vi "Q Vision_2017 Object Calcs.vi"(4 "Threshhold":i32=50, 6 "ColorMask Low/High":u8[][](array[numeric])=[[0, 100], [200, 255], [170, 230]], 7 "ColorSpace":T1, 8 "error in (no error)":errorcluster, 10 "Image in":T3) -> (0 "error out":errorcluster, 3 "Object Params out":T2 {"Deg_Up" format="%.2f"; "Deg_Rt" format="%.2f"; "Dist_ft" format="%.1f"})   [LabVIEW 2016]
uses:
  <vilib>/vision/Image Controls.llb/IMAQ Image.ctl
  Typedefs/typedef_cluster_Object Params.ctl
  Quick Vision/Typedefs/typedef_enum_ColorSpace.ctl
panel:
  out "B/W Image":i16[][](graph)
  out "Image Pixels (U32)":u32[][](array[numeric]) format="%08x"
  out "B/W Image_Object":i16[][](graph)
  # "R"
  # "G"
  # "B"
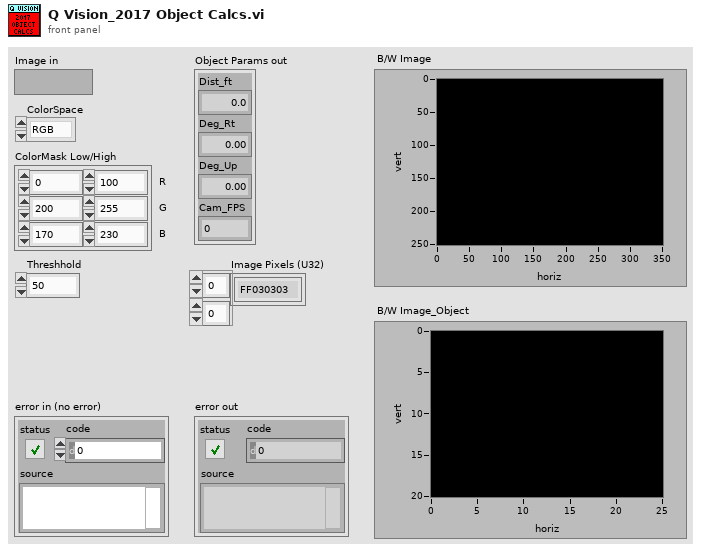
[diagram p1: front panel]
types:
  T1 = typedef "typedef_enum_ColorSpace.ctl" = enum16{"RGB", "HSL"}
  T2 = typedef "typedef_cluster_Object Params.ctl" = cluster{"Dist_ft":dbl, "Deg_Rt":dbl, "Deg_Up":dbl, "Cam_FPS":dbl}
  T3 = typedef "IMAQ Image.ctl" = refnum<image>
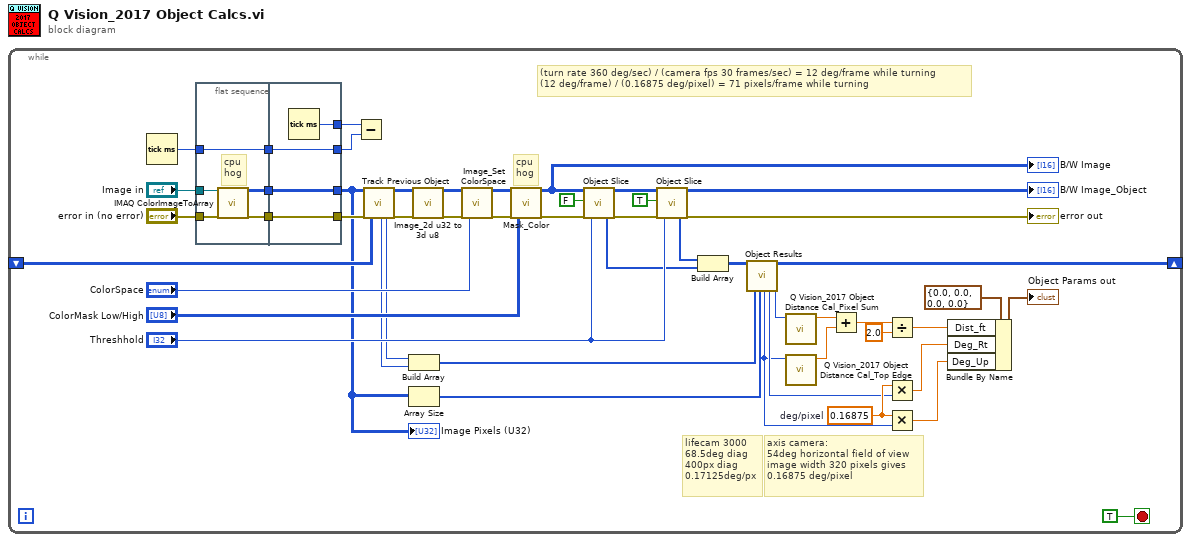
[diagram p0: block diagram]
diagram:
  n1 = while {
    shift-right: [w12] -> _
    shift-left: _ -> [w23]
    stop <- TRUE stop-if-true
    w31 = 0.16875  # deg/pixel
    # "lifecam 3000\n68.5deg diag\n400px diag\n0.17125deg/px"
    # "(turn rate 360 deg/sec) / (camera fps 30 frames/sec) = 12 deg/frame while turning\n(12 deg/frame) / (0.16875 deg/pixel) = 71 pixels/frame while turning"
    # "axis camera:\n54deg horizontal field of view\nimage width 320 pixels gives\n0.16875 deg/pixel"
    # "cpu\nhog"
    n2 = Tick Count (ms)() -> (millisecond timer value=w39:u32)
    n3 = flat-sequence {
      tunnel: [w55] -> w49
      tunnel: [w53] -> w48
      tunnel: [w54] -> w47
      tunnel: w39 -> [w53]
      tunnel: "Image in" -> [w52]
      tunnel: "error in (no error)" -> [w51]
      tunnel: [w57] -> w22
      tunnel: [w58] -> w33
      tunnel: [w59] -> w20
      tunnel: w49 -> [w59]
      tunnel: w48 -> [w58]
      tunnel: w47 -> [w57]
      tunnel: [w56] -> w34
      frame #0 {
        # "cpu\nhog"
        n4 = call "IMAQ ColorImageToArray"("Image"=w52, "error in (no error)"=w51) -> ("Image Pixels (U32)"=w55:u32[][], "error out"=w54:errorcluster)  [unwired: 2 in, 1 out]
      }
      frame #1 {
        n5 = Tick Count (ms)() -> (millisecond timer value=w56:u32)
      }
    }
    n6 = Subtract(x=w34, y=w33) -> ()  [unwired: 1 out]
    n7 = call "Track Previous Object.vi"("Image_2d_u32 in"=w20, "error in (no error)"=w22, "Prev. Object Start/Stop/Sum"=w23) -> ("Col Offset"=w17:i32, "Row Offset"=w18:i32, "Image_2d_u32 out"=w24:u32[][], "error out"=w21:errorcluster)  [unwired: 13 in]
    n8 = Build Array(w18, w17) -> (w8:i32[])
    n9 = Array Size(array=w20) -> (size(s)=w9:i32[])
    n10 = call "Image_2d u32 to 3d u8.vi"("Image_2d_u32"=w24, "error in (no error)"=w21) -> ("Image_3d_u8"=w45:u8[][][], "error out"=w43:errorcluster)  [unwired: 16 in]
    n11 = call "Image_Set ColorSpace.vi"("Image_3d"=w45, "error in (no error)"=w43, "ColorSpace"="ColorSpace") -> ("Image_3d_ColorSpace"=w44:u8[][][], "error out"=w46:errorcluster)  [unwired: 14 in, 1 out]
    n12 = call "Mask_Color.vi"("Image_3d"=w44, "error in (no error)"=w46, "ColorMask Low/High"="ColorMask Low/High") -> ("Image_2d"=w30:i16[][], "error out"=w42:errorcluster)  [unwired: 14 in, 1 out]
    "B/W Image" <- w30
    n13 = call "Object Slice.vi"("Image_2d"=w30, "Slice Rows(T)/Cols(F)"=FALSE, "error in (no error)"=w42, "Threshhold"="Threshhold") -> ("Object Start/Stop/Sum"=w15:i32[], "Image_2d_Slice"=w40:i16[][], "error out"=w27:errorcluster)  [unwired: 13 in]
    n14 = call "Object Slice.vi"("Image_2d"=w40, "Slice Rows(T)/Cols(F)"=TRUE, "error in (no error)"=w27, "Threshhold"="Threshhold") -> ("Object Start/Stop/Sum"=w16:i32[], "Image_2d_Slice"=→"B/W Image_Object":i16[][], "error out"=→"error out":errorcluster)  [unwired: 13 in]
    n15 = Build Array(w16, w15) -> (w13:i32[][])
    n16 = call "Object Results.vi"("Object Start/Stop/Sum in"=w13, "Offset rows,cols"=w8, "Image rows,cols"=w9) -> ("Pixels Up"=w5:i32, "Pixels Rt"=w10:i32, "Object Start/Stop/Sum out"=w12:i32[][], "Pixel Sum"=w11:i32)  [unwired: 13 in]
    n17 = call "Q Vision_2017 Object Distance Cal_Pixel Sum.vi"("Pixel Sum"=w11) -> ("Distance (ft)"=w6:dbl)  [unwired: 10 in]
    n18 = call "Q Vision_2017 Object Distance Cal_Top Edge.vi"("Pixels Up"=w5) -> ("Distance (ft)"=w3:dbl)  [unwired: 10 in]
    n19 = Add(x=w6, y=w3) -> (x+y=w4:dbl)
    n20 = Divide(x=w4, y=2.0) -> (x/y=w2:dbl)
    n21 = Multiply(x=w31, y=w10) -> (x*y=w14:dbl)
    n22 = Multiply(x=w31, y=w5) -> (x*y=w32:dbl)
    n23 = Bundle By Name(cluster=T2 {"Dist_ft"=0.0, "Deg_Rt"=0.0, "Deg_Up"=0.0, "Cam_FPS"=0.0} ("Object Params out"), "Dist_ft"=w2, "Deg_Rt"=w14, "Deg_Up"=w32) -> (→"Object Params out":T2)
    "Image Pixels (U32)" <- w20
  }
